vi "MathConstants.vi"(1 "Constant Name":T1) -> (0 "Constant Value":dbl)   [LabVIEW 2015]
uses:
  <userlib>/836-Library/CheezyMath/MathConstantsNames.ctl
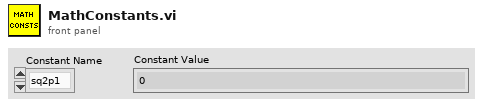
[diagram p1: front panel]
types:
  T1 = typedef "MathConstantsNames.ctl" = enum16{"sq2p1", "sq2m1", "p4", "p3", "p2", "p1", "p0", "q4", "q3", "q2", "q1", "q0", "PIO2"}
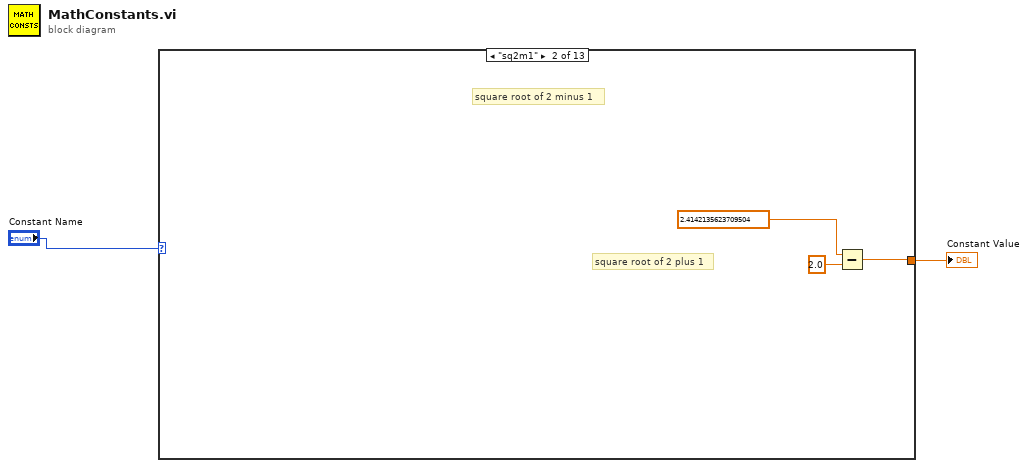
[diagram p0: block diagram]
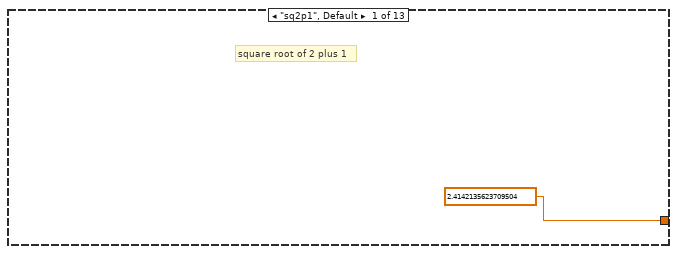
[diagram p2: hidden frame]
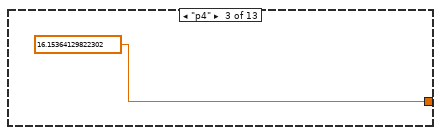
[diagram p3: hidden frame]
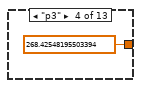
[diagram p4: hidden frame]
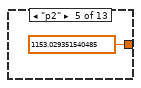
[diagram p5: hidden frame]
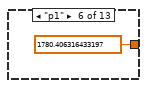
[diagram p6: hidden frame]
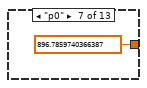
[diagram p7: hidden frame]
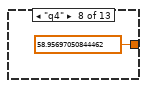
[diagram p8: hidden frame]
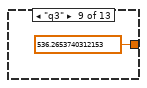
[diagram p9: hidden frame]
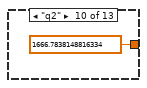
[diagram p10: hidden frame]
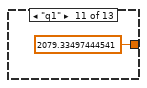
[diagram p11: hidden frame]
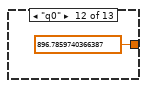
[diagram p12: hidden frame]
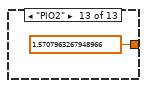
[diagram p13: hidden frame]
diagram:
  n1 = case shown="\"sq2m1\"" "Constant Name" {
    tunnel: [2.4142135623709504 w6 16.15364129822302 268.42548195503394 1153.029351540485 1780.406316433197 896.7859740366387 58.95697050844462 536.2653740312153 1666.7838148816334 2079.33497444541 896.7859740366387 1.5707963267948966] -> w2
    frame "sq2p1", Default {
      # "square root of 2 plus 1"
    }
    frame "sq2m1" {
      # "square root of 2 plus 1"
      # "square root of 2 minus 1"
      n2 = Subtract(x=2.4142135623709504, y=2.0) -> (x-y=w6:dbl)
    }
    frame "p4" {
    }
    frame "p3" {
    }
    frame "p2" {
    }
    frame "p1" {
    }
    frame "p0" {
    }
    frame "q4" {
    }
    frame "q3" {
    }
    frame "q2" {
    }
    frame "q1" {
    }
    frame "q0" {
    }
    frame "PIO2" {
    }
  }
  "Constant Value" <- w2
